vi "PyrometerSetpoint.vi"() -> ()   [LabVIEW 2018]
uses:
  C:/Users/bowenm/Git/Acquisition/Instruments/ImagingPyrometer/Kineses/Thorlabs.MotionControl.Controls.dll
  Kineses/Thorlabs.MotionControl.Controls.dll
  C:/Users/bowenm/Git/Acquisition/Instruments/ImagingPyrometer/Kineses/ThorLabs.MotionControl.KCube.DCServoCLI.dll
  Kineses/ThorLabs.MotionControl.KCube.DCServoCLI.dll
  Global Variables.vi
  <vilib>/Utility/file.llb/Read Delimited Spreadsheet (string).vi
  <instrlib>/Thorlabs_FW102C/Thorlabs_FW102C.lvlib
panel:
  in  "Stop":bool
  in  "Set":bool
  out "Position Error":bool
  out "NDFW102C out":i32
  in  "NDFW Serial Port":string="COM5"
  out "tdms file out":refnum<k34>
  out "RFW wls":string[](array[string])=["1000", "850", "800", "700", "650", "600"]
  out "TFW wls":string[](array[string])=["900", "850", "800", "750", "700", "600"]
  in  "Tab Control":enum32{"400-700nm", "700-1100nm"}(tab)
  in  "VisTFW Wavelength":u16(ring) caption="Wavelength 1" items=["600", "700"]
  in  "VisRFW Wavelength":u16(ring) caption="Wavelength 2" items=["600", "650", "700"]
  in  "NIRRFW Wavelengths":u16(ring) caption="Wavelength 2" items=["700", "800", "850", "1000"]
  in  "NIRTFW Wavelengths":u16(ring) caption="Wavelength 1" items=["700", "750", "800", "850", "900"]
  out "NDFs":dbl[](array[numeric])=[0.0, 0.2, 0.4, 0.5, 0.6, 1.0]
  in  "NeutralDensityFilter":u16(ring) items=["0", "0.2", "0.4", "0.5", "0.6", "1"]
  out "RFW102C out":i32=1
  in  "RFW Serial Port":string="COM3"
  out "error out":errorcluster
  out "TFW102C out":i32
  in  "TFW Serial Port":string="COM4"
  out "MotorMoving":bool
  out "Device":refnum<k24>
  in  "KCubeDCServoControl":refnum<k24>(container)
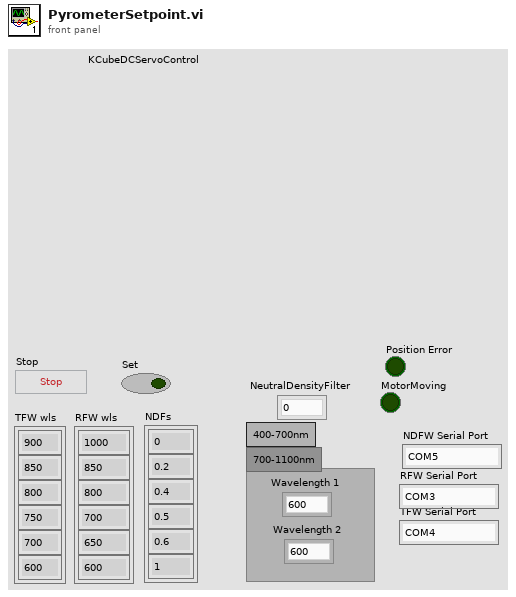
[diagram p1: front panel]
types:
  T1 = enum16{"open", "open or create", "create or replace", "create", "open (read-only)"}
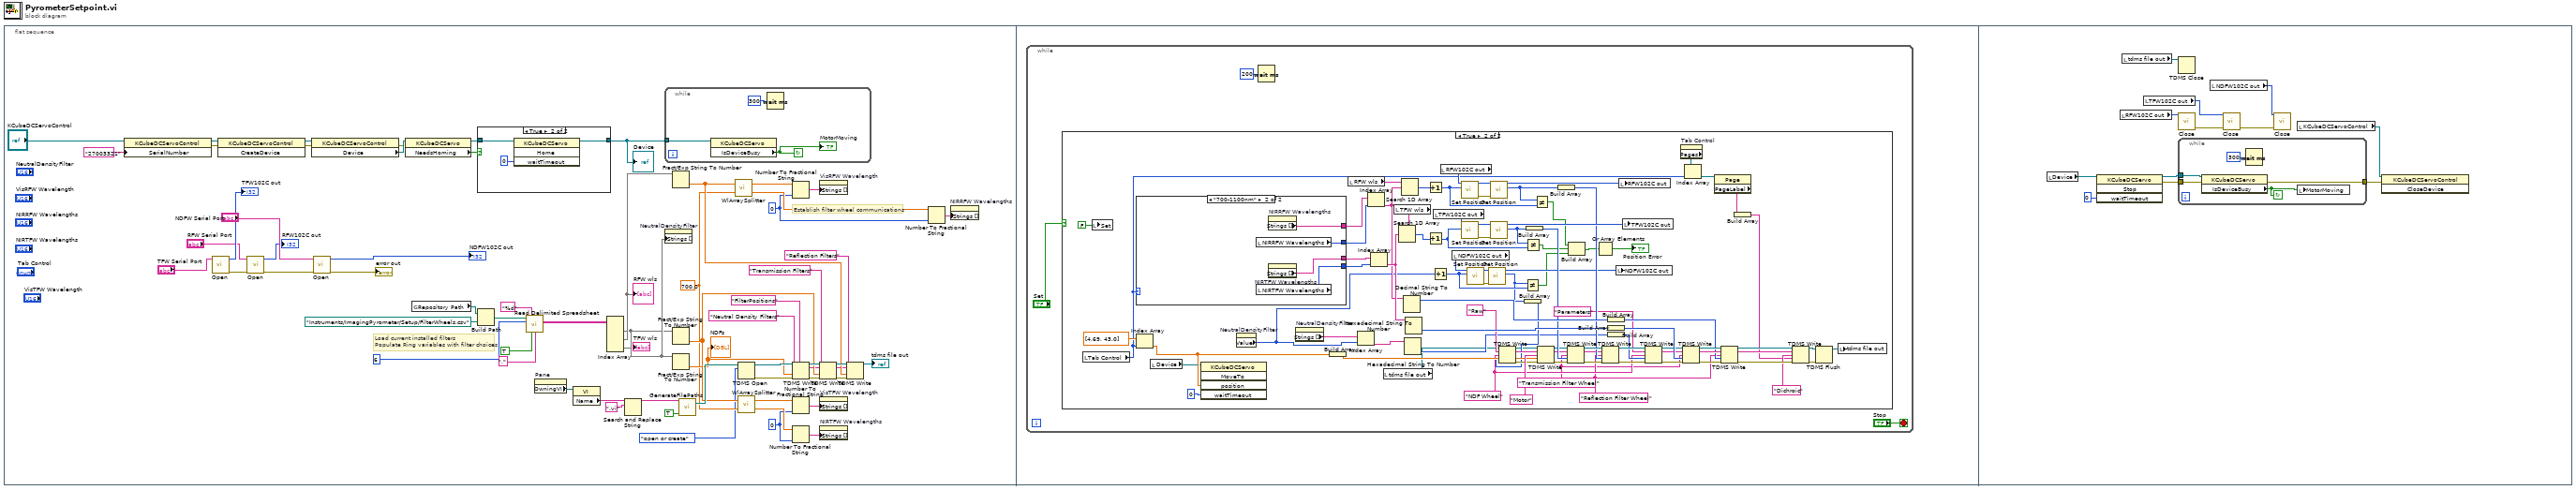
[diagram p0: block diagram]
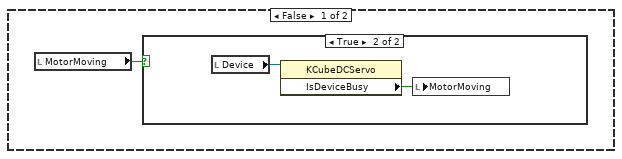
[diagram p3: hidden frame]
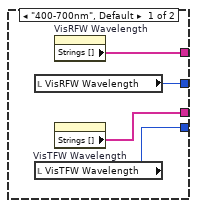
[diagram p5: hidden frame]
diagram:
  n1 = flat-sequence {
    frame #0 {
      w8 = i16 0 ("precision (6)")
      w9 = 700.0 ("Cutoff Wavelength")
      w10 = i16 0 ("precision (6)")
      # "Load current installed filters\nPopulate Ring variables with filter choices"
      # "Establish filter wheel communications"
      n2 = property class="KCubeDCServoControl"(reference="KCubeDCServoControl", "SerialNumber"="27003321") -> (reference out=w25:refnum<k24>, error out=w24:errorcluster)  [unwired: 1 in]
      n3 = call <instrlib>:"Open.vi"("Serial Port"="TFW Serial Port") -> ("error out"=w29:errorcluster, "FW102C out"=→"TFW102C out":i32)  [unwired: 8 in, 1 out]
      n4 = invoke class="KCubeDCServoControl" method="CreateDevice"(reference=w25, error in=w24) -> (reference out=w23:refnum<k24>, error out=w22:errorcluster)  [unwired: 1 in, 1 out]
      n5 = call <instrlib>:"Open.vi"("error in (no error)"=w29, "Serial Port"="RFW Serial Port") -> ("error out"=w28:errorcluster, "FW102C out"=→"RFW102C out":i32)  [unwired: 7 in, 1 out]
      n6 = property class="KCubeDCServoControl"(reference=w23, error in=w22) -> (error out=w20:errorcluster, "Device"=w21:refnum<k24>)  [unwired: 1 out]
      n7 = call <instrlib>:"Open.vi"("error in (no error)"=w28, "Serial Port"="NDFW Serial Port") -> ("error out"=→"error out":errorcluster, "FW102C out"=→"NDFW102C out":i32)  [unwired: 7 in, 1 out]
      n8 = property class="KCubeDCServo"(reference=w21, error in=w20) -> (reference out=w19:refnum<k24>, "NeedsHoming"=w18:bool)  [unwired: 1 out]
      n9 = global read "Global Variables.vi" "Repository Path"() -> (w35:path)
      n10 = case shown="True" w18 {
        tunnel: w19 -> [w69 w72]
        tunnel: [w69 w71] -> w17
        frame False {
        }
        frame True {
          n11 = invoke class="KCubeDCServo" method="Home"(reference=w72, "waitTimeout"=0) -> (reference out=w71:refnum<k24>)  [unwired: 2 in, 3 out]
        }
      }
      "Device" <- w17
      n12 = Build Path(base path=w35, name or relative path=path "Instruments/ImagingPyrometer/Setup/FilterWheels.csv" ("vi path")) -> (appended path=w34:path)
      n13 = call-poly <vilib>:"Read Delimited Spreadsheet.vi"("file path (dialog if empty)"=w34, "format (%s)"="%d", "number of rows (all:-1)"=6, "transpose? (F)"=TRUE, "delimiter (\\t)"="," ("delimiter (\\t)")) -> ("all rows"=w40:string[][])  [unwired: 5 in, 5 out]
      n14 = property on="Pane" class="Pane"() -> ("OwningVI"=w59:refnum<vi>)  [unwired: 2 in, 2 out]
      n15 = property class="VI"(reference=w59) -> ("Name"=w61:string)  [unwired: 1 in, 2 out]
      n16 = Index Array(array=w40) -> (element #1=w41:string[], element #2=w42:string[], element #3=w47:string[])  [unwired: 6 in]
      "TFW wls" <- w41
      "RFW wls" <- w42
      n17 = Search and Replace String(input string=w61, search string=".vi") -> (result string=w60:string)  [unwired: 6 in, 3 out]
      n18 = while {
        tunnel: w17 -> [w66]
        stop <- w68 continue-if-true
        n19 = property class="KCubeDCServo"(reference=w66) -> ("IsDeviceBusy"=w68:bool)  [unwired: 1 in, 2 out]
        "MotorMoving" <- w68
        n20 = Wait (ms)(milliseconds to wait=u32 300) -> ()  [unwired: 1 out]
      }
      n21 = property on="NeutralDensityFilter" class="Ring (strict)"("Strings []"=w47) -> ()  [unwired: 2 in, 2 out]
      n22 = Fract/Exp String To Number(string=w42) -> (number=w52:dbl[])  [unwired: 3 in, 1 out]
      n23 = Fract/Exp String To Number(string=w41) -> (number=w50:dbl[])  [unwired: 3 in, 1 out]
      n24 = Fract/Exp String To Number(string=w47) -> (number=w48:dbl[])  [unwired: 3 in, 1 out]
      "NDFs" <- w48
      n25 = call "GenerateFilePaths.vi"("Logfile? (F)"=TRUE ("Logfile?"), "Device Name"=w60) -> ("Path"=w62:path)  [unwired: 3 in]
      n26 = call "WlArraySplitter.vi"("Cutoff Wavelength"=w9, "Wavelength Array"=w52) -> ("Higher Wavelengths"=w44:dbl[], "Lower Wavelengths"=w43:dbl[])
      n27 = TDMS Open(10:T1."open or create" ("operation (0:open)"), 11:w62) -> (0:w54:errorcluster, 3:w53:refnum<k34>)  [unwired: 5 in]
      n28 = call "WlArraySplitter.vi"("Cutoff Wavelength"=w9, "Wavelength Array"=w50) -> ("Higher Wavelengths"=w39:dbl[], "Lower Wavelengths"=w38:dbl[])
      n29 = Number To Fractional String(number=w43, precision (6)=w8) -> (F-format string=w46:string[])  [unwired: 2 in]
      n30 = TDMS Write(0:w53, 5:"FilterPositions" ("group name in (Untitled)"), 7:"Neutral Density Filters", 9:w48, 11:w54) -> (4:w55:refnum<k34>, 6:w49:string, 15:w56:errorcluster)  [unwired: 1 in, 1 out]
      n31 = Number To Fractional String(number=w38, precision (6)=w10) -> (F-format string=w36:string[])  [unwired: 2 in]
      n32 = Number To Fractional String(number=w39, precision (6)=w10) -> (F-format string=w37:string[])  [unwired: 2 in]
      n33 = property on="VisRFW Wavelength" class="Ring (strict)"("Strings []"=w46) -> ()  [unwired: 2 in, 2 out]
      n34 = TDMS Write(0:w55, 5:w49, 7:"Transmission Filters", 9:w50, 11:w56) -> (4:w58:refnum<k34>, 6:w51:string, 15:w57:errorcluster)  [unwired: 1 in, 1 out]
      n35 = property on="VisTFW Wavelength" class="Ring (strict)"("Strings []"=w36) -> ()  [unwired: 2 in, 2 out]
      n36 = property on="NIRTFW Wavelengths" class="Ring (strict)"("Strings []"=w37) -> ()  [unwired: 2 in, 2 out]
      n37 = TDMS Write(0:w58, 5:w51, 7:"Reflection Filters", 9:w52, 11:w57) -> (4:→"tdms file out":refnum<k34>)  [unwired: 1 in, 3 out]
      n38 = Number To Fractional String(number=w44, precision (6)=w8) -> (F-format string=w45:string[])  [unwired: 2 in]
      n39 = property on="NIRRFW Wavelengths" class="Ring (strict)"("Strings []"=w45) -> ()  [unwired: 2 in, 2 out]
    }
    frame #1 {
      n40 = while {
        stop <- "Stop" stop-if-true
        n41 = case shown="True" "Set" {
          frame False {
            n42 = local read "MotorMoving"() -> (w76:bool)
            n43 = case shown="True" w76 {
              frame False {
              }
              frame True {
                n44 = local read "Device"() -> (w77:refnum<k24>)
                n45 = property class="KCubeDCServo"(reference=w77) -> ("IsDeviceBusy"=w78:bool)  [unwired: 1 in, 2 out]
                n46 = local write "MotorMoving"(w78) -> ()
              }
            }
          }
          frame True {
            w86 = "NDF Wheel"
            w83 = "Reflection Filter Wheel"
            w82 = "Transmission Filter Wheel"
            n47 = local read "Tab Control"() -> (w111:enum32{"400-700nm", "700-1100nm"})
            n48 = local write "Set"(FALSE ("Set")) -> ()
            n49 = case shown="\"700-1100nm\"" w111 {
              tunnel: [w166 w170] -> w129
              tunnel: [w168 w173] -> w128
              tunnel: [w167 w171] -> w131
              tunnel: [w169 w172] -> w130
              frame "400-700nm", Default {
                n50 = local read "VisRFW Wavelength"() -> (w168:u16)
                n51 = local read "VisTFW Wavelength"() -> (w169:u16)
                n52 = property on="VisRFW Wavelength" class="Ring (strict)"() -> ("Strings []"=w166:string[])  [unwired: 2 in, 2 out]
                n53 = property on="VisTFW Wavelength" class="Ring (strict)"() -> ("Strings []"=w167:string[])  [unwired: 2 in, 2 out]
              }
              frame "700-1100nm" {
                n54 = local read "NIRRFW Wavelengths"() -> (w173:u16)
                n55 = local read "NIRTFW Wavelengths"() -> (w172:u16)
                n56 = property on="NIRRFW Wavelengths" class="Ring (strict)"() -> ("Strings []"=w170:string[])  [unwired: 2 in, 2 out]
                n57 = property on="NIRTFW Wavelengths" class="Ring (strict)"() -> ("Strings []"=w171:string[])  [unwired: 2 in, 2 out]
              }
            }
            n58 = Index Array(array=dbl[] [4.69, 43.0], index=w111) -> (element=w114:dbl)
            n59 = local read "Device"() -> (w113:refnum<k24>)
            n60 = invoke class="KCubeDCServo" method="MoveTo"(reference=w113, "position"=w114, "waitTimeout"=0) -> ()  [unwired: 2 in, 5 out]
            n61 = property on="NeutralDensityFilter" class="Ring (strict)"() -> ("Value"=w80:u16)  [unwired: 2 in, 2 out]
            n62 = property on="NeutralDensityFilter" class="Ring (strict)"() -> ("Strings []"=w90:string[])  [unwired: 2 in, 2 out]
            n63 = Build Array(w114) -> (w112:dbl[])
            n64 = local read "RFW wls"() -> (w159:string[])
            n65 = Index Array(array=w90, index=w80) -> (element=w88:string)
            n66 = Index Array(array=w129, index=w128) -> (element=w145:string)
            n67 = Index Array(array=w131, index=w130) -> (element=w151:string)
            n68 = local read "tdms file out"() -> (w84:refnum<k34>)
            n69 = local read "TFW wls"() -> (w154:string[])
            n70 = Search 1D Array(1D array=w154, element=w151) -> (index of element=w155:i32)  [unwired: 1 in]
            n71 = Search 1D Array(1D array=w159, element=w145) -> (index of element=w158:i32)  [unwired: 1 in]
            n72 = Decimal String To Number(string=w145) -> (offset past number=w144:i32)  [unwired: 2 in, 1 out]
            n73 = Hexadecimal String To Number(string=w88) -> (number=w87:u32)  [unwired: 2 in, 1 out]
            n74 = Hexadecimal String To Number(string=w151) -> (number=w150:u32)  [unwired: 2 in, 1 out]
            n75 = Increment(x=w158) -> (x+1=w164:i32)
            n76 = Increment(x=w155) -> (x+1=w165:i32)
            n77 = Increment(x=w80) -> (x+1=w105:u16)
            n78 = local read "TFW102C out"() -> (w156:i32)
            n79 = local read "RFW102C out"() -> (w157:i32)
            n80 = local read "NDFW102C out"() -> (w107:i32)
            n81 = call <instrlib>:"Set Position.vi"("Position"=w164, "FW102C in"=w157) -> ("error out"=w162:errorcluster, "FW102C out"=w163:i32)  [unwired: 8 in]
            n82 = call <instrlib>:"Set Position.vi"("Position"=w165, "FW102C in"=w156) -> ("error out"=w161:errorcluster, "FW102C out"=w160:i32)  [unwired: 8 in]
            n83 = call <instrlib>:"Set Position.vi"("Position"=w105, "FW102C in"=w107) -> ("error out"=w109:errorcluster, "FW102C out"=w108:i32)  [unwired: 8 in]
            n84 = call <instrlib>:"Get Position.vi"("error in (no error)"=w109, "FW102C in"=w108) -> ("Position"=w92:i32, "FW102C out"=w106:i32)  [unwired: 7 in, 1 out]
            n85 = call <instrlib>:"Get Position.vi"("error in (no error)"=w162, "FW102C in"=w163) -> ("Position"=w118:i32, "FW102C out"=w152:i32)  [unwired: 7 in, 1 out]
            n86 = call <instrlib>:"Get Position.vi"("error in (no error)"=w161, "FW102C in"=w160) -> ("Position"=w117:i32, "FW102C out"=w153:i32)  [unwired: 7 in, 1 out]
            n87 = Build Array(w92) -> (w91:i32[])
            n88 = TDMS Write(0:w84, 5:"Raw", 7:w86, 9:w91) -> (4:w85:refnum<k34>, 6:w94:string, 15:w95:errorcluster)  [unwired: 2 in, 1 out]
            n89 = Not Equal?(x=w92, y=w105) -> (x != y?=w104:bool)
            n90 = Not Equal?(x=w117, y=w165) -> (x != y?=w79:bool)
            n91 = Build Array(w117) -> (w122:i32[])
            n92 = Not Equal?(x=w118, y=w164) -> (x != y?=w81:bool)
            n93 = TDMS Write(0:w85, 5:w94, 7:"Motor", 9:w112, 11:w95) -> (4:w120:refnum<k34>, 6:w121:string, 15:w123:errorcluster)  [unwired: 1 in, 1 out]
            n94 = Build Array(w118) -> (w125:i32[])
            n95 = TDMS Write(0:w120, 5:w121, 7:w82, 9:w122, 11:w123) -> (4:w126:refnum<k34>, 6:w124:string, 15:w127:errorcluster)  [unwired: 1 in, 1 out]
            n96 = Build Array(w81, w79, w104) -> (w103:bool[])
            n97 = Or Array Elements(Boolean array=w103) -> (logical OR=→"Position Error":bool)
            n98 = TDMS Write(0:w126, 5:w124, 7:w83, 9:w125, 11:w127) -> (4:w98:refnum<k34>, 15:w100:errorcluster)  [unwired: 1 in, 2 out]
            n99 = Build Array(w144) -> (w143:i32[])
            n100 = Build Array(w150) -> (w149:u32[])
            n101 = Build Array(w87) -> (w89:u32[])
            n102 = local write "NDFW102C out"(w106) -> ()
            n103 = local write "RFW102C out"(w152) -> ()
            n104 = local write "TFW102C out"(w153) -> ()
            n105 = TDMS Write(0:w98, 5:"Parameters", 7:w86, 9:w89, 11:w100) -> (4:w101:refnum<k34>, 6:w97:string, 15:w99:errorcluster)  [unwired: 1 in, 1 out]
            n106 = property on="Tab Control" class="TabCtl (strict)"() -> ("Pages"=w138:refnum<vi>[])  [unwired: 2 in, 2 out]
            n107 = TDMS Write(0:w101, 5:w97, 7:w82, 9:w149, 11:w99) -> (4:w148:refnum<k34>, 6:w147:string, 15:w146:errorcluster)  [unwired: 1 in, 1 out]
            n108 = Index Array(array=w138, index=w111) -> (element=w137:refnum<vi>)
            n109 = property class="Page"(reference=w137) -> ("PageLabel"=w136:string)  [unwired: 1 in, 2 out]
            n110 = TDMS Write(0:w148, 5:w147, 7:w83, 9:w143, 11:w146) -> (4:w142:refnum<k34>, 6:w141:string, 15:w140:errorcluster)  [unwired: 1 in, 1 out]
            n111 = Build Array(w136) -> (w135:string[])
            n112 = TDMS Write(0:w142, 5:w141, 7:"Dichroic", 9:w135, 11:w140) -> (4:w133:refnum<k34>, 15:w132:errorcluster)  [unwired: 1 in, 2 out]
            n113 = TDMS Flush(4:w132, 7:w133) -> (3:w134:refnum<k34>)  [unwired: 1 out]
            n114 = local write "tdms file out"(w134) -> ()
          }
        }
        n115 = Wait (ms)(milliseconds to wait=u32 200) -> ()  [unwired: 1 out]
      }
    }
    frame #2 {
      n116 = local read "Device"() -> (w175:refnum<k24>)
      n117 = invoke class="KCubeDCServo" method="Stop"(reference=w175, "waitTimeout"=0) -> (reference out=w178:refnum<k24>, error out=w177:errorcluster)  [unwired: 2 in, 2 out]
      n118 = local read "RFW102C out"() -> (w182:i32)
      n119 = local read "tdms file out"() -> (w183:refnum<k34>)
      n120 = local read "TFW102C out"() -> (w181:i32)
      n121 = TDMS Close(11:w183) -> ()  [unwired: 1 in, 2 out]
      n122 = call <instrlib>:"Close.vi"("FW102C in"=w182) -> ("error out"=w180:errorcluster)  [unwired: 10 in]
      n123 = while {
        tunnel: w178 -> [w190]
        tunnel: [w187] -> w176
        tunnel: w177 -> [w186]
        stop <- w188 continue-if-true
        n124 = property class="KCubeDCServo"(reference=w190, error in=w186) -> (error out=w187:errorcluster, "IsDeviceBusy"=w188:bool)  [unwired: 1 out]
        n125 = Wait (ms)(milliseconds to wait=u32 300) -> ()  [unwired: 1 out]
        n126 = local write "MotorMoving"(w188) -> ()
      }
      n127 = local read "NDFW102C out"() -> (w185:i32)
      n128 = call <instrlib>:"Close.vi"("error in (no error)"=w180, "FW102C in"=w181) -> ("error out"=w184:errorcluster)  [unwired: 9 in]
      n129 = call <instrlib>:"Close.vi"("error in (no error)"=w184, "FW102C in"=w185) -> ()  [unwired: 9 in, 1 out]
      n130 = local read "KCubeDCServoControl"() -> (w179:refnum<k24>)
      n131 = invoke class="KCubeDCServoControl" method="CloseDevice"(reference=w179, error in=w176) -> ()  [unwired: 1 in, 3 out]
    }
  }
